vi "Build Server.vi"(8 "Error In":errorcluster, 10 "Lines":T1[](array[typedef]), 11 "OPC UA server refnum in":refnum<k21>) -> (0 "Error Out":errorcluster, 3 "OPC UA server refnum out":refnum<k21>)   [LabVIEW 2013, in "OPC UA runtime.lvclass"]
doc: "Build OPC UA Server Folder/Item Hierarchy"
uses:
  OPC UA runtime.lvclass
  configuration/Line.ctl
  <vilib>/NI/Tag Bus Module Framework/channel/TBM channel.lvclass
  configuration/OPC UA Data Type.ctl
  <vilib>/opcua/NI OPC UA Server.lvlib
  configuration/OPC UA configuration.lvclass
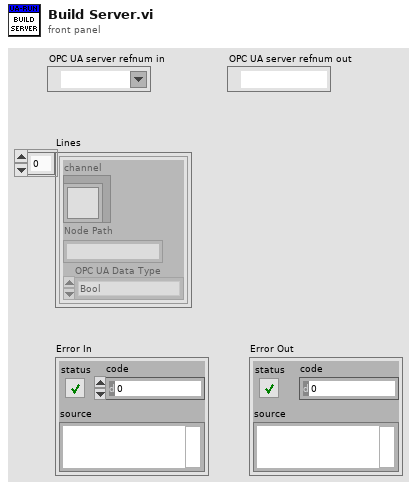
[diagram p1: front panel]
types:
  T1 = typedef "OPC UA configuration.lvclass/Line.ctl" = cluster{"channel":refnum<class "TBM channel.lvclass">, "Node Path":string, "OPC UA Data Type":T2}
  T2 = typedef "OPC UA configuration.lvclass/OPC UA Data Type.ctl" = enum16{"Bool", "SByte", "Byte", "Int16", "UInt16", "Int32", "UInt32", "Int64", "UInt64", "Float", "Double", "String", "DateTime", "ByteString", "Bool Array", "SByte Array", "Byte Array", "Int16 Array", "UInt16 Array", "Int32 Array", "UInt32 Array", "Int64 Array", "UInt64 Array", "Float Array", "Double Array", "String Array", "DateTime Array", "ByteString Array"}
  T3 = cluster{"name":string, "data type":u16, "access level":u16, "description":string}
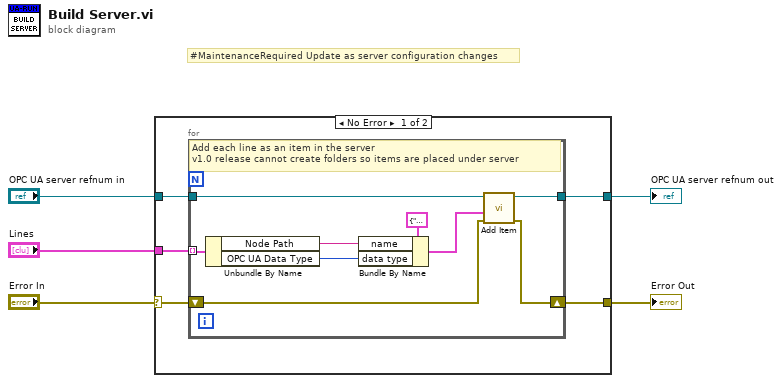
[diagram p0: block diagram]
diagram:
  # "#MaintenanceRequired Update as server configuration changes"
  n1 = case shown="No Error" "Error In" {
    selector: "Error In" -> [w7 w21]
    tunnel: "OPC UA server refnum in" -> [w10 w20]
    tunnel: "Lines" -> [w9 _]
    tunnel: [w8 w21] -> w3
    tunnel: [w6 w20] -> w1
    frame No Error {
      n2 = for {
        tunnel: w10 -> [w19]
        tunnel: w9 -> [w18] mode=indexing
        shift-right: [w12] -> w8
        shift-left: w7 -> [w13]
        tunnel: [w11] -> w6
        # "Add each line as an item in the server\nv1.0 release cannot create folders so items are placed under server"
        n3 = Unbundle By Name(w18) -> ("Node Path"=w16:string, "OPC UA Data Type"=w15:T2)
        n4 = Bundle By Name(cluster=T3 {"name"="", "data type"=1, "access level"=1, "description"=""} ("item"), "name"=w16, "data type"=w15) -> (w14:T3)
        n5 = call <vilib>:"Add Item.vi"("error in (no error)"=w13, "item"=w14, "OPC UA server refnum in"=w19) -> ("error out"=w12:errorcluster, "OPC UA server refnum out"=w11:refnum<k21>)  [unwired: 5 in, 1 out]
      }
    }
    frame Error {
    }
  }
  "OPC UA server refnum out" <- w1
  "Error Out" <- w3
